vi "Measurement Logic.vi"() -> ()   [LabVIEW 2021, in "Keysight 34461A DMM Measurement.lvlib"]
uses:
  Keysight 34461A DMM Measurement.lvlib
  <vilib>/Plug-In SDKs/Measurements/Measure Call Context/Measure Call Context.lvclass
  <vilib>/Plug-In SDKs/Clients/Session Management V1/Session Reservation/Session Reservation.lvclass
  Measurement Configuration.ctl
  Measurement Results.ctl
  subVIs/Keysight 34461A Function.ctl
panel:
  out "error out":errorcluster
  out "measure call context out":refnum<class "Measure Call Context.lvclass">
  in  "measure call context in":refnum<class "Measure Call Context.lvclass">
  out "measurement results":T1
  in  "measurement configuration":T2={"pin_name"="", "measurement_type"=enum."DC Voltage", "auto_range"=FALSE, "manual_range"=0.0, "resolution_digits"=0.0}
  in  "error in":errorcluster
  # "Measurement Type: value"
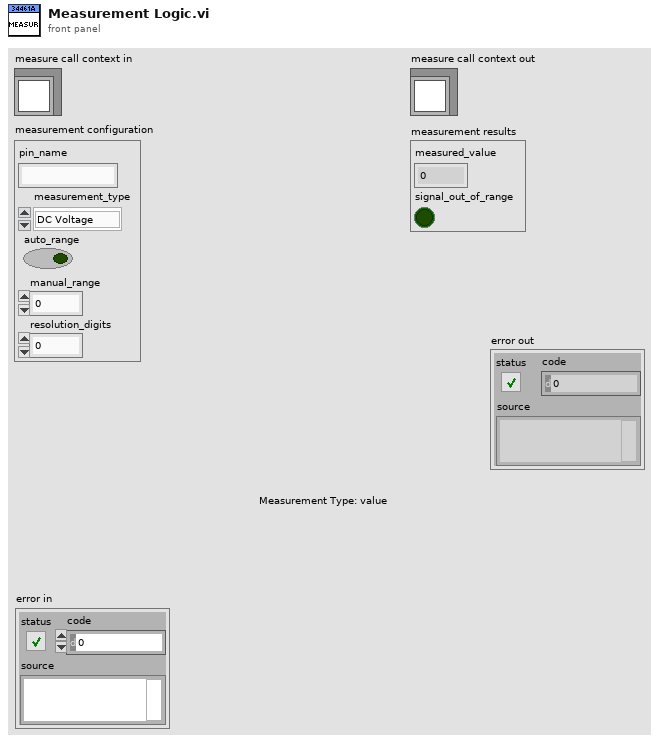
[diagram p1: front panel]
types:
  T1 = typedef "Keysight 34461A DMM Measurement.lvlib/Measurement Results.ctl" = cluster{"measured_value":dbl, "signal_out_of_range":bool}
  T2 = typedef "Keysight 34461A DMM Measurement.lvlib/Measurement Configuration.ctl" = cluster{"pin_name":string, "measurement_type":T3, "auto_range":bool, "manual_range":dbl, "resolution_digits":dbl}
  T3 = typedef "Keysight 34461A DMM Measurement.lvlib/Keysight 34461A Function.ctl" = enum32{"Continuity", "AC Current", "DC Current", "Diode Checking", "Frequency", "4 - Wire Resistance", "Period", "2 - Wire Resistance", "Temperature", "AC Voltage", "DC Voltage", "VDC:VDC Ratio", "Capacitance"}
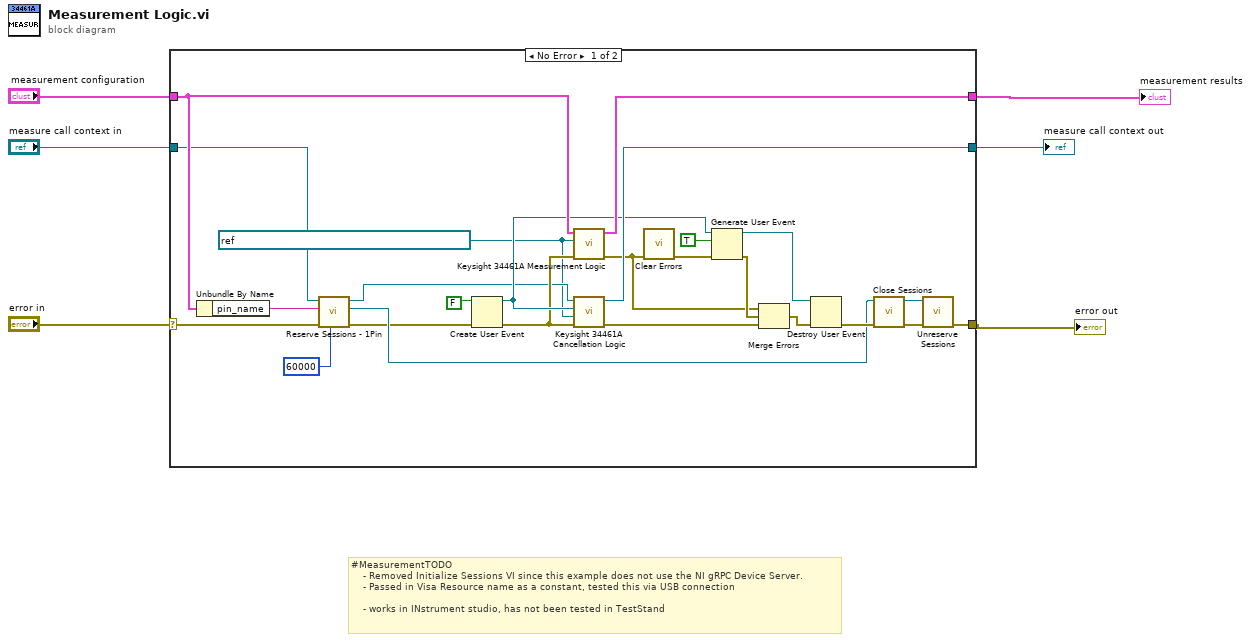
[diagram p0: block diagram]
diagram:
  # "#MeasurementTODO\n    - Removed Initialize Sessions VI since this example does not use the NI gRPC Device Server.\n    - Passed in Visa Resource name as a constant, tested this via USB connection\n\n    - works in INstrument studio, has not been tested in TestStand"
  n1 = case shown="No Error" "error in" {
    selector: "error in" -> [w17 w33]
    tunnel: "measure call context in" -> [w18 w32]
    tunnel: [w13 w33] -> w1
    tunnel: "measurement configuration" -> [w30 _]
    tunnel: [w31 _] -> w2
    tunnel: [w29 w32] -> w4
    frame No Error {
      w9 = refnum<visa-resource-name> "USB0::0x2A8D::0x1301::MY53215615::INSTR" ("VISA resource name out")
      n2 = Unbundle By Name(w30) -> ("pin_name"=w16:string)
      n3 = call <vilib>:"Reserve Sessions - 1Pin.vi"("timeout (ms)"=60000 ("timeout in milliseconds"), "error in"=w17, "pin or relay name"=w16, "measurement context in"=w18) -> ("error out"=w7:errorcluster, "session reservation out"=w8:refnum<class "Session Reservation.lvclass">, "measurement context out"=w14:refnum<class "Measure Call Context.lvclass">)  [unwired: 5 in]
      n4 = Create User Event(user event datatype=FALSE ("measurement complete"), error in=w7) -> (user event=w25:refnum<user-event>, error out=w23:errorcluster)
      n5 = call "Keysight 34461A Measurement Logic.vi"("error in (no error)"=w23, "session"=w9, "measurement configuration"=w30) -> ("error out"=w19:errorcluster, "measurement results"=w31:T1)  [unwired: 7 in]
      n6 = call "Keysight 34461A Cancellation Logic.vi"("error in (no error)"=w23, "session"=w9, "measurement complete"=w25, "MeasurementContext in"=w14) -> ("error out"=w28:errorcluster, "MeasurementContext out"=w29:refnum<class "Measure Call Context.lvclass">)  [unwired: 6 in]
      n7 = call <vilib>:"Clear Errors.vi"("error in (no error)"=w19) -> ("error out"=w20:errorcluster)  [unwired: 5 in, 1 out]
      n8 = Generate User Event(user event=w25, event data cluster=TRUE ("event data"), error in=w20) -> (user event out=w21:refnum<user-event>, error out=w24:errorcluster)  [unwired: 1 in]
      n9 = Merge Errors(w19, w24, w28) -> (w22:errorcluster)
      n10 = Destroy User Event(user event=w21, error in=w22) -> (error out=w12:errorcluster)
      n11 = call <vilib>:"Close Sessions.vi"("error in"=w12, "session reservation in"=w8) -> ("error out"=w11:errorcluster, "session reservation out"=w10:refnum<class "Session Reservation.lvclass">)  [unwired: 8 in]
      n12 = call <vilib>:"Unreserve Sessions.vi"("error in"=w11, "session reservation in"=w10) -> ("error out"=w13:errorcluster)  [unwired: 9 in]
    }
    frame Error {
    }
  }
  "measurement results" <- w2
  "measure call context out" <- w4
  "error out" <- w1
